vi "Read Attributes.vi"(11 "Set HVAC Control Msg":refnum<class "Set HVAC Control Msg.lvclass">) -> (2 "Payload":cluster{"HVAC_Control":T1})   [LabVIEW 2018, in "Device Communication and Control Abstract Actor.lvlib" / "Set HVAC Control Msg.lvclass"]
uses:
  Set HVAC Control Msg.lvclass
  <vilib>/ORNL/CSEISMIC DDS/CSEISMIC DDS Base/Data Types/HVAC_Control.ctl
  <vilib>/ORNL/CSEISMIC DDS/CSEISMIC DDS Base/Data Types/Controls/DeviceID.ctl
  <vilib>/ORNL/CSEISMIC DDS/CSEISMIC DDS Base/Data Types/Controls/ControlMode.ctl
  Set HVAC Control Msg.lvclass/Set HVAC Control Msg.ctl
  <vilib>/ORNL/CSEISMIC DDS/CSEISMIC DDS Base/CSEISMIC DDS.lvclass
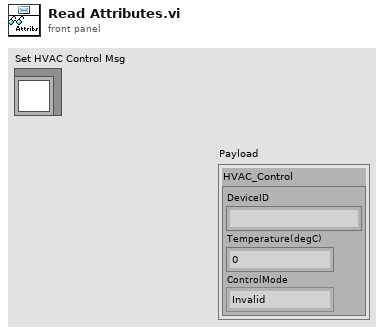
[diagram p1: front panel]
types:
  T1 = typedef "CSEISMIC DDS.lvlib/CSEISMIC DDS.lvclass/HVAC_Control.ctl" = cluster{"DeviceID":T2, "Temperature(degC)":dbl, "ControlMode":T3}
  T2 = typedef "CSEISMIC DDS.lvlib/CSEISMIC DDS.lvclass/DeviceID.ctl" = string
  T3 = typedef "CSEISMIC DDS.lvlib/CSEISMIC DDS.lvclass/ControlMode.ctl" = enum32{"Invalid", "Cooling", "Heating"}
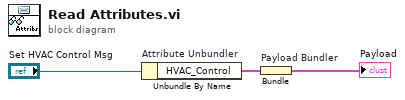
[diagram p0: block diagram]
diagram:
  n1 = Unbundle By Name "Attribute Unbundler"("Set HVAC Control Msg") -> ("HVAC_Control"=w1:T1)
  n2 = Bundle "Payload Bundler"("HVAC_Control"=w1) -> (→"Payload":cluster{"HVAC_Control":T1})  [unwired: 1 in]
